vi "Mouse Move.vi"(8 "error in (no error)":errorcluster, 10 "y":i32, 11 "x":i32) -> (0 "error out":errorcluster)   [LabVIEW 2020, in "MacroAssert.lvlib"]
uses:
  MacroAssert.lvlib
  user32.dll
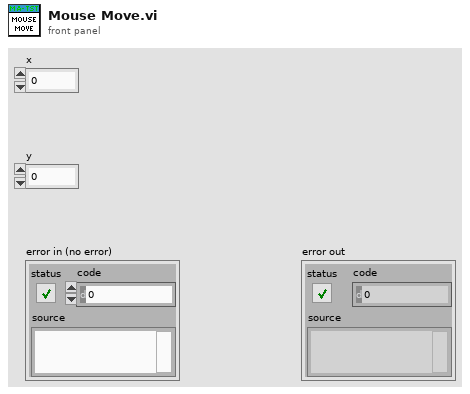
[diagram p1: front panel]
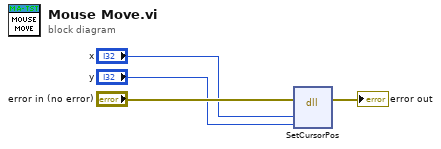
[diagram p0: block diagram]
diagram:
  n1 = dll-call lib="user32.dll" fn="SetCursorPos"(error in="error in (no error)", "x"="x", "y"="y") -> (error out=→"error out":errorcluster)  [unwired: 5 in, 1 out]
